vi "Request Check-In.vi"(0 "Guest Manager UI in":refnum<class "Guest Manager UI.lvclass">, 11 "error in (no error)":errorcluster) -> (4 "Guest Manager UI out":refnum<class "Guest Manager UI.lvclass">, 15 "error out":errorcluster)   [LabVIEW 2023, in "Guest Manager UI.lvlib" / "Guest Manager UI.lvclass"]
uses:
  Guest Manager UI.lvclass
  C:/Program Files/National Instruments/LabVIEW 2023/vi.lib/ActorFramework/Actor/Actor.lvclass
  <vilib>/ActorFramework/Actor/Actor.lvclass/Actor.ctl
  Guest Manager UI.lvclass/Guest Manager UI.ctl
  Guest Manager UI Messages/Verify and Check-in Msg/Verify and Check-in Msg.lvclass/Verify and Check-in Msg.ctl
  <vilib>/ActorFramework/Message Enqueuer/Message Enqueuer.lvclass/Message Enqueuer.ctl
  <vilib>/ActorFramework/Message Enqueuer/Enqueue.vi
  Guest Manager UI Messages/Verify and Check-in Msg/Verify and Check-in Msg.lvclass
  C:/Program Files/National Instruments/LabVIEW 2023/vi.lib/ActorFramework/Message/Message.lvclass
  <vilib>/ActorFramework/Message Priority Queue/Priority Enqueue.vi
  <vilib>/ActorFramework/Actor/Actor.lvclass
  Utilities/Utilities.lvlib
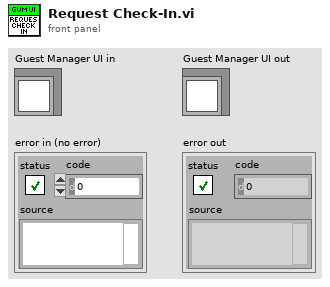
[diagram p1: front panel]
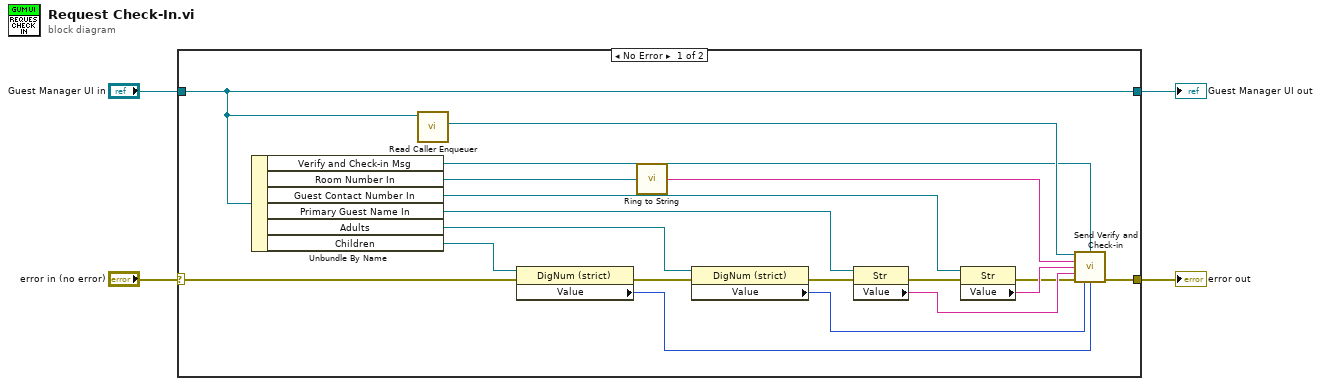
[diagram p0: block diagram]
diagram:
  n1 = case shown="No Error" "error in (no error)" {
    selector: "error in (no error)" -> [w23 w25]
    tunnel: [w17 w25] -> w3
    tunnel: [w22 w24] -> w1
    tunnel: "Guest Manager UI in" -> [w22 w24]
    frame No Error {
      n2 = Unbundle By Name(w22) -> ("Verify and Check-in Msg"=w15:refnum<class "Verify and Check-in Msg.lvclass">, "Room Number In"=w21:refnum<vi>, "Guest Contact Number In"=w7:refnum<vi>, "Primary Guest Name In"=w11:refnum<vi>, "Adults"=w18:refnum<vi>, "Children"=w20:refnum<vi>)
      n3 = call <vilib>:"Read Caller Enqueuer.vi"("Actor"=w22) -> ("Caller Enqueuer"=w16:refnum<class "Message Enqueuer.lvclass">)  [unwired: 10 in]
      n4 = property class="DigNum (strict)"(reference=w20, error in=w23) -> (error out=w19:errorcluster, "Value"=w13:u32)  [unwired: 1 out]
      n5 = call "Ring to String.vi"("Ring Ctrl Ref"=w21) -> ("Output String"=w14:string)
      n6 = property class="DigNum (strict)"(reference=w18, error in=w19) -> (error out=w10:errorcluster, "Value"=w12:u32)  [unwired: 1 out]
      n7 = property class="Str"(reference=w11, error in=w10) -> (error out=w8:errorcluster, "Value"=w9:string)  [unwired: 1 out]
      n8 = property class="Str"(reference=w7, error in=w8) -> (error out=w5:errorcluster, "Value"=w6:string)  [unwired: 1 out]
      n9 = call "Send Verify and Check-in.vi"("Message Enqueuer"=w16, "Message Type"=w15, "Room No"=w14, "Guest Contact Number"=w6, "Primary Guest Name"=w9, "error in (no error)"=w5, "Adults"=w12, "Children"=w13) -> ("error out"=w17:errorcluster)  [unwired: 6 in, 1 out]
    }
    frame Error {
    }
  }
  "error out" <- w3
  "Guest Manager UI out" <- w1
